vi "LockIn_#2_data.vi"() -> (0 "String":string)   [LabVIEW 2016]
uses:
  Instrument_Setup.vi
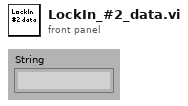
[diagram p1: front panel]
types:
  T1 = cluster{"sensitivity\n2nV/fA":i32, "dyn reserve\n(low noise:2)":i16, "ref. phase":ext, "automeasure":bool}
  T2 = cluster{"time constant\n(10 µs : 0) ":i32, "slope (6 dB/oct)":i32}
  T3 = cluster{"input":u16, "ground":bool, "couple":bool}
  T4 = cluster{"off. & exp.":u16, "offset":dbl, "expand":u16}
  T5 = cluster{"ref. source":bool, "osc.harm# ":u16, "osc. freq":ext, "osc. ampl.":ext, "ref. trigger":u16}
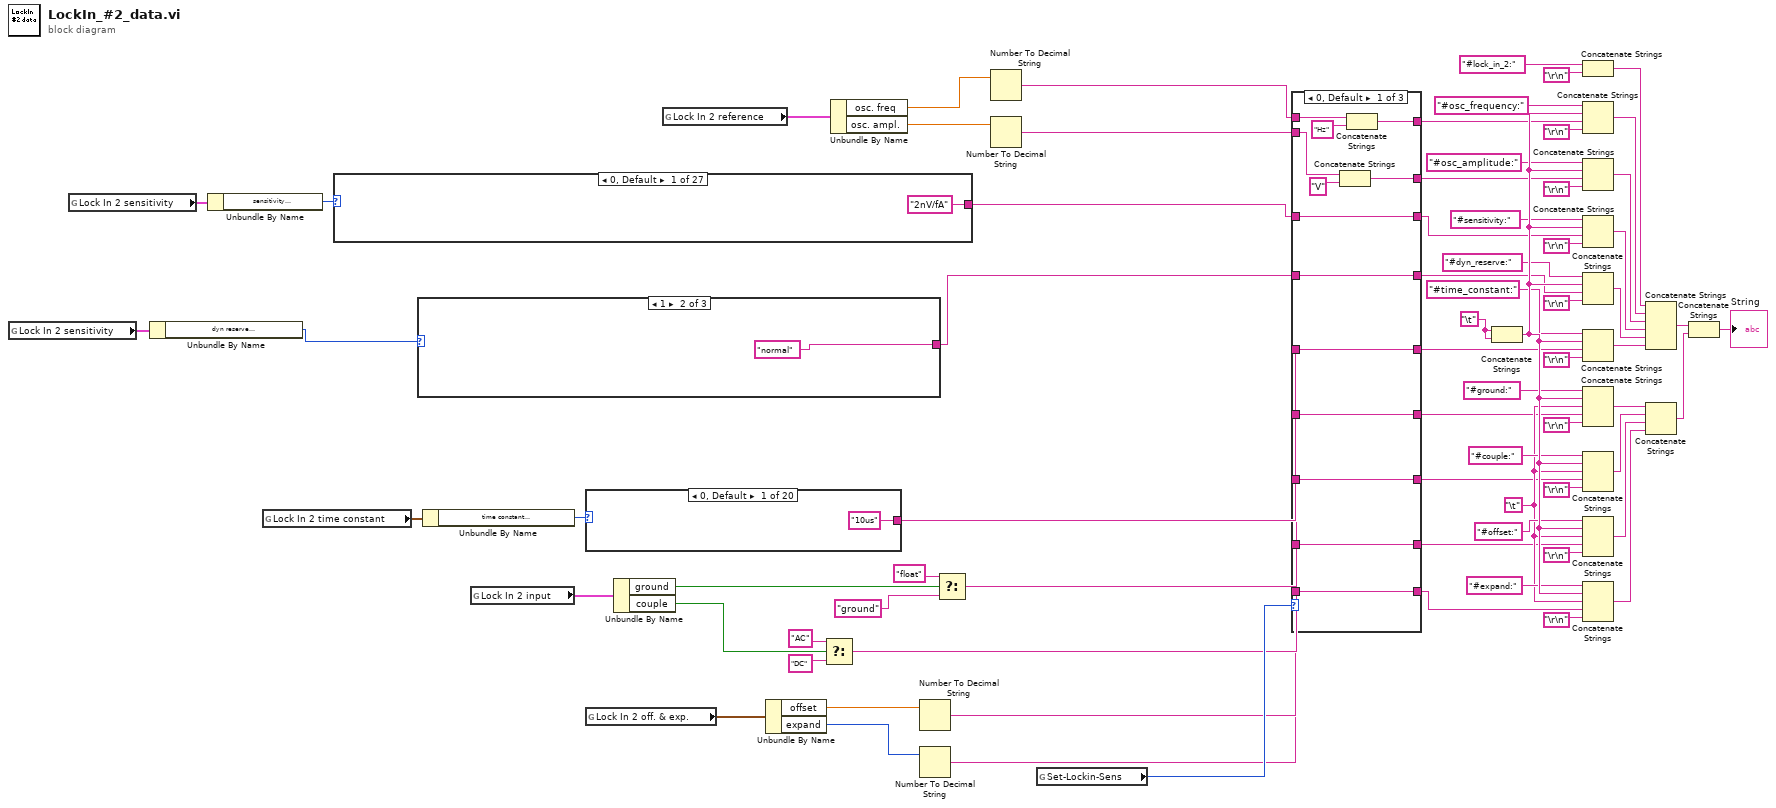
[diagram p0: block diagram]
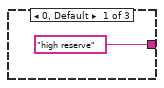
[diagram p2: hidden frame]
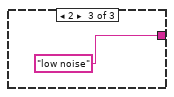
[diagram p3: hidden frame]
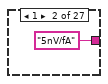
[diagram p4: hidden frame]
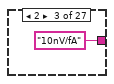
[diagram p5: hidden frame]
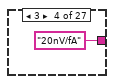
[diagram p6: hidden frame]
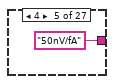
[diagram p7: hidden frame]
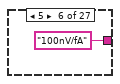
[diagram p8: hidden frame]
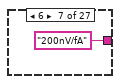
[diagram p9: hidden frame]
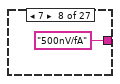
[diagram p10: hidden frame]
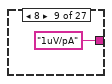
[diagram p11: hidden frame]
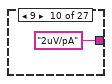
[diagram p12: hidden frame]
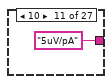
[diagram p13: hidden frame]
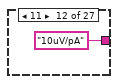
[diagram p14: hidden frame]
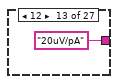
[diagram p15: hidden frame]
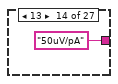
[diagram p16: hidden frame]
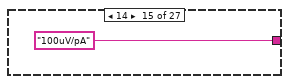
[diagram p17: hidden frame]
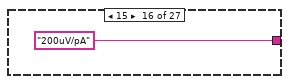
[diagram p18: hidden frame]
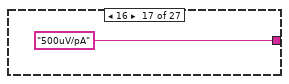
[diagram p19: hidden frame]
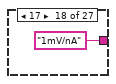
[diagram p20: hidden frame]
diagram:
  w24 = "\t"
  w73 = "\t"
  n1 = global read "Instrument_Setup.vi" "Lock In 2 sensitivity"() -> (w39:T1)
  n2 = global read "Instrument_Setup.vi" "Lock In 2 sensitivity"() -> (w34:T1)
  n3 = Unbundle By Name(w39) -> ("dyn reserve\n(low noise:2)"=w1:i16)
  n4 = Unbundle By Name(w34) -> ("sensitivity\n2nV/fA"=w20:i32)
  n5 = global read "Instrument_Setup.vi" "Lock In 2 time constant"() -> (w41:T2)
  n6 = case shown="0, Default" w20 {
    tunnel: ["2nV/fA" "5nV/fA" "10nV/fA" "20nV/fA" "50nV/fA" "100nV/fA" "200nV/fA" "500nV/fA" "1uV/pA" "2uV/pA" "5uV/pA" "10uV/pA" "20uV/pA" "50uV/pA" "100uV/pA" "200uV/pA" "500uV/pA" "1mV/nA" "2mV/nA" "5mV/nA" "10mV/nA" "20mV/nA" "50mV/nA" "100mV/nA" "200mV/nA" "500mV/nA" "1V/uA"] -> w3
    frame 0, Default {
    }
    frame 1 {
    }
    frame 2 {
    }
    frame 3 {
    }
    frame 4 {
    }
    frame 5 {
    }
    frame 6 {
    }
    frame 7 {
    }
    frame 8 {
    }
    frame 9 {
    }
    frame 10 {
    }
    frame 11 {
    }
    frame 12 {
    }
    frame 13 {
    }
    frame 14 {
    }
    frame 15 {
    }
    frame 16 {
    }
    frame 17 {
    }
    frame 18 {
    }
    frame 19 {
    }
    frame 20 {
    }
    frame 21 {
    }
    frame 22 {
    }
    frame 23 {
    }
    frame 24 {
    }
    frame 25 {
    }
    frame 26 {
    }
  }
  n7 = case shown="1" w1 {
    tunnel: ["high reserve" "normal" "low noise"] -> w2
    frame 0, Default {
    }
    frame 1 {
    }
    frame 2 {
    }
  }
  n8 = Unbundle By Name(w41) -> ("time constant\n(10 µs : 0)"=w21:i32)
  n9 = global read "Instrument_Setup.vi" "Lock In 2 input"() -> (w47:T3)
  n10 = case shown="0, Default" w21 {
    tunnel: ["10us" "30us" "100us" "300us" "1ms" "3ms" "10ms" "30ms" "100ms" "300ms" "1s" "3s" "10s" "30s" "100s" "300s" "1ks" "3ks" "10ks" "30ks"] -> w19
    frame 0, Default {
    }
    frame 1 {
    }
    frame 2 {
    }
    frame 3 {
    }
    frame 4 {
    }
    frame 5 {
    }
    frame 6 {
    }
    frame 7 {
    }
    frame 8 {
    }
    frame 9 {
    }
    frame 10 {
    }
    frame 11 {
    }
    frame 12 {
    }
    frame 13 {
    }
    frame 14 {
    }
    frame 15 {
    }
    frame 16 {
    }
    frame 17 {
    }
    frame 18 {
    }
    frame 19 {
    }
  }
  n11 = global read "Instrument_Setup.vi" "Lock In 2 off. & exp."() -> (w55:T4)
  n12 = Unbundle By Name(w47) -> ("ground"=w48:bool, "couple"=w49:bool)
  n13 = global read "Instrument_Setup.vi" "Lock In 2 reference"() -> (w30:T5)
  n14 = Unbundle By Name(w55) -> ("offset"=w56:dbl, "expand"=w57:u16)
  n15 = Select(t="AC", s=w49, f="DC") -> (s? t:f=w14:string)
  n16 = Unbundle By Name(w30) -> ("osc. freq"=w31:ext, "osc. ampl."=w32:ext)
  n17 = Number To Decimal String(number=w56) -> (decimal integer string=w12:string)  [unwired: 1 in]
  n18 = Number To Decimal String(number=w57) -> (decimal integer string=w10:string)  [unwired: 1 in]
  n19 = Select(t="float", s=w48, f="ground") -> (s? t:f=w16:string)
  n20 = Number To Decimal String(number=w31) -> (decimal integer string=w8:string)  [unwired: 1 in]
  n21 = Number To Decimal String(number=w32) -> (decimal integer string=w6:string)  [unwired: 1 in]
  n22 = global read "Instrument_Setup.vi" "Set-Lockin-Sens"() -> (w22:u16)
  n23 = case shown="0, Default" w22 {
    tunnel: w19 -> [w137 w145 w153]
    tunnel: w3 -> [w136 w144 w152]
    tunnel: [w137 w145 w153] -> w18
    tunnel: [w136 w144 w152] -> w17
    tunnel: w16 -> [w135 w143 w151]
    tunnel: [w135 w143 w151] -> w15
    tunnel: w14 -> [w134 w142 w150]
    tunnel: [w134 w142 w150] -> w13
    tunnel: w12 -> [w133 w141 w149]
    tunnel: [w133 w141 w149] -> w11
    tunnel: w10 -> [w132 w140 w148]
    tunnel: [w132 w140 w148] -> w9
    tunnel: w8 -> [w131 _ _]
    tunnel: [w129 w138 w146] -> w7
    tunnel: w6 -> [w128 _ _]
    tunnel: [w126 w138 w146] -> w5
    tunnel: w2 -> [w125 w139 w147]
    tunnel: [w125 w139 w147] -> w4
    frame 0, Default {
      n24 = Concatenate Strings(w128, "V" ("String")) -> (w126:string)
      n25 = Concatenate Strings(w131, "Hz" ("String")) -> (w129:string)
    }
    frame 2 {
      w138 = "manual"
    }
    frame 1 {
      w146 = "auto"
    }
  }
  n26 = Concatenate Strings(w73, w73) -> (w74:string)
  n27 = Concatenate Strings("#lock_in_2:", "\r\n") -> (w29:string)
  n28 = Concatenate Strings("#osc_frequency:", w74, w7, "\r\n") -> (w61:string)
  n29 = Concatenate Strings("#osc_amplitude:" ("String"), w74, w5, "\r\n") -> (w62:string)
  n30 = Concatenate Strings("#sensitivity:" ("String"), w74, w17, "\r\n") -> (w63:string)
  n31 = Concatenate Strings("#dyn_reserve:" ("String"), w74, w4, "\r\n") -> (w64:string)
  n32 = Concatenate Strings("#time_constant:" ("String"), w74, w18, "\r\n") -> (w65:string)
  n33 = Concatenate Strings("#ground:" ("String"), w74, w24, w15, "\r\n") -> (w66:string)
  n34 = Concatenate Strings("#couple:" ("String"), w74, w24, w13, "\r\n") -> (w67:string)
  n35 = Concatenate Strings("#offset:" ("String"), w74, w24, w11, "\r\n") -> (w68:string)
  n36 = Concatenate Strings("#expand:" ("String"), w74, w24, w9, "\r\n") -> (w69:string)
  n37 = Concatenate Strings(w29, w61, w62, w63, w64, w65) -> (w70:string)
  n38 = Concatenate Strings(w66, w67, w68, w69) -> (w71:string)
  n39 = Concatenate Strings(w70, w71) -> (→"String":string)
